vi "LS340Monitor.vi"() -> ()   [LabVIEW 2019]
uses:
  Equipment/Lake Shore Cryotronics 340/Lake Shore Cryotronics 340.lvlib
  Global/Global Variables/Data_Display_global.vi
  Instrument_Setup.vi
panel:
  in  "stop 2":bool
  in  "VISA session 2":refnum<visa-resource-name>="GPIB0::12::INSTR"
  out "SP kleiner als":dbl
  out "Temperature (K)":dbl=291.191
  in  "stop":bool
  in  "VISA session":refnum<visa-resource-name>="GPIB0::12::INSTR"
  out "Temperature":cluster{dbl[], dbl[]}(graph)={[452.667759], [291.191]}
  out "Heater Power":cluster{dbl[], dbl[]}(graph)={[452.667759], [0.0]}
  out "Heater Power (%)":dbl
  out "Heater (%)":dbl(slide) scale=0.0..100.0
  out "Setpoint ITC (K)":dbl=300.0
  out "Offset new SP":dbl
  out "Heater Range":dbl
  out "P (Gain)":dbl
  out "I (Reset)":dbl
  out "D (Rate)":dbl
  in  "Update every [ms]":dbl min=0.0 max=10000.0 step=500.0
  out "HeaterTableLS340.txt":string caption="PID Table"
  in  "Pfad zu HeaterTable":path=path "D:/Cryostat Software/CryoTUM-V1.0/sub_vi-s/Heater Tables/HeaterTableLS340.txt"
  # "0: Off\n1: 10mW\n2: 100mW\n3: 1.0W\n4: 10W"
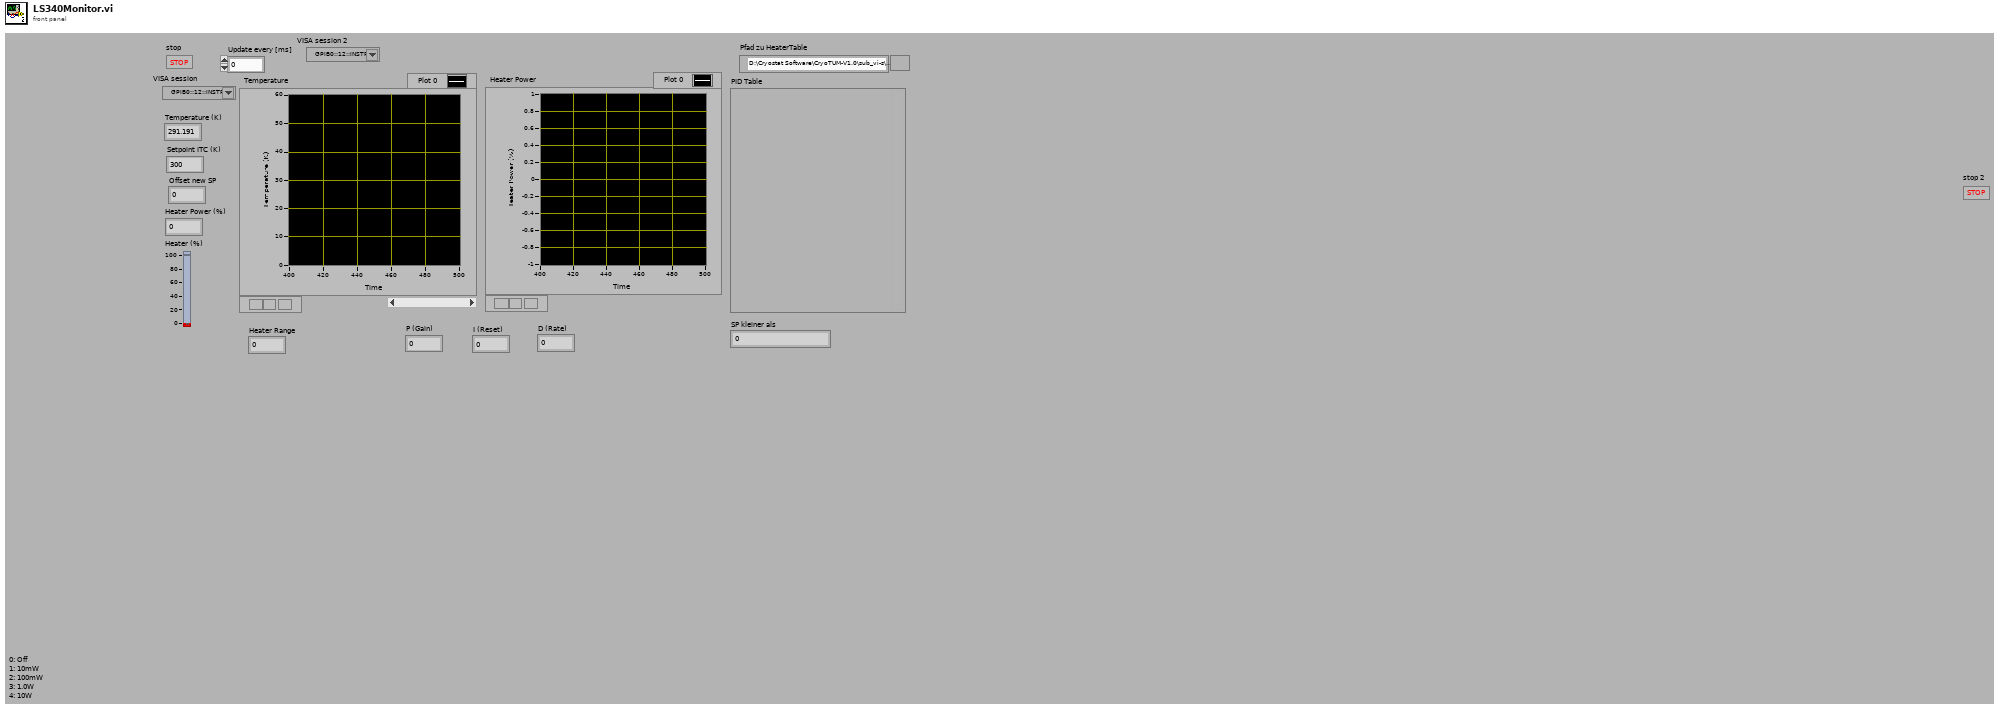
[diagram p1: front panel]
types:
  T1 = enum16{"open", "replace", "create", "open or create", "replace or create", "replace or create with confirmation"}
  T2 = typedef "ITCVersion.ctl" = enum16{"ITC502", "ITC503", "ITC601"}
  T3 = cluster{"Version":T2, "ControlTITC":i8, "ControlTCh":i8, "SampleTITC":i8, "SampleTCh":i8, "Instrument address":cluster{"Com Port":i32, "ISOBUS Address":i32, "GPIB Address":i16, "Communication":enum16{"RS232", "ISOBUS", "GPIB", "Gateway"}}}
  T4 = cluster{"Com Port":i32, "ISOBUS Address":i32, "GPIB Address":i16, "Communication":enum16{"RS232", "ISOBUS", "GPIB", "Gateway"}}
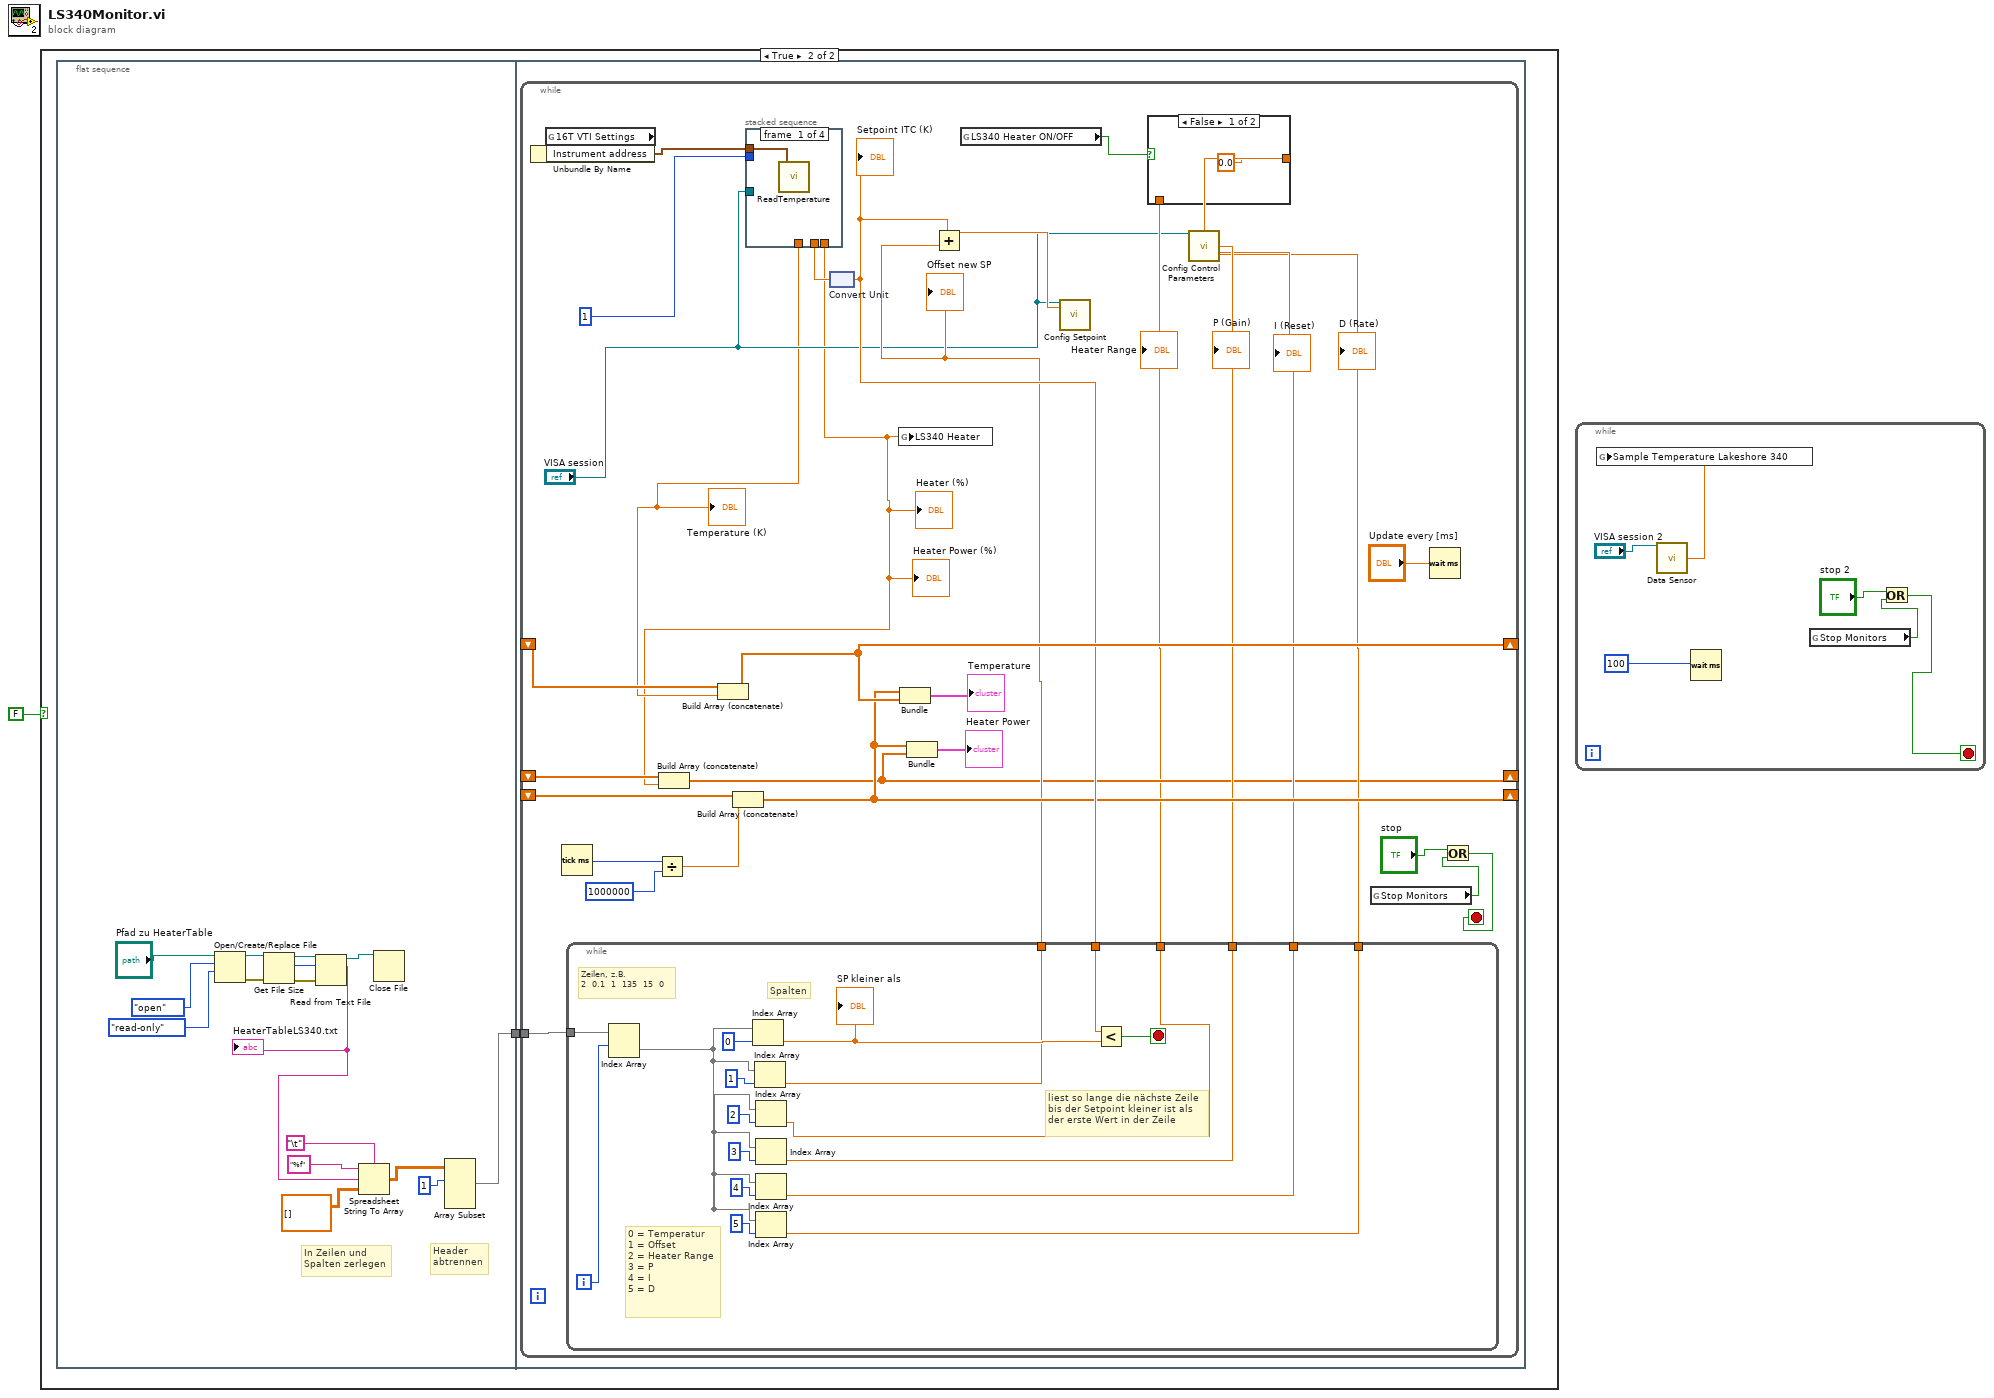
[diagram p0: block diagram]
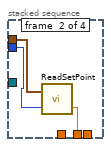
[diagram p3: hidden frame]
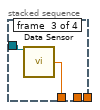
[diagram p4: hidden frame]
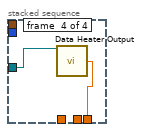
[diagram p5: hidden frame]
diagram:
  n1 = case shown="True" FALSE {
    frame False {
    }
    frame True {
      n2 = flat-sequence {
        tunnel: [w3] -> w2
        tunnel: w2 -> [w19]
        frame #0 {
          # "In Zeilen und \nSpalten zerlegen"
          # "Header\nabtrennen"
          n3 = Open/Create/Replace File(file path (use dialog)="Pfad zu HeaterTable", operation (0:open)=T1."open", access (0:read/write)=enum16{"read/write", "read-only", "write-only"}."read-only") -> (refnum out=w13:refnum<file>, error out=w15:errorcluster)  [unwired: 3 in, 1 out]
          n4 = Get File Size(file=w13, error in=w15) -> (refnum out=w12:refnum<file>, size (in bytes)=w8:i64, 0:w14:errorcluster)
          n5 = Read from Text File(file (use dialog)=w12, count=w8, error in=w14) -> (refnum out=w11:refnum<file>, text=w7:string)  [unwired: 1 in, 2 out]
          "HeaterTableLS340.txt" <- w7
          n6 = Spreadsheet String To Array(delimiter (Tab)="\t", format string="%f", spreadsheet string=w7, array type (2D Dbl)=dbl[][] []) -> (array=w6:dbl[][])
          n7 = Close File(refnum=w11) -> ()  [unwired: 1 in, 2 out]
          n8 = Array Subset(array=w6, index (row)=1) -> (w3:dbl[][])  [unwired: 3 in]
        }
        frame #1 {
          n9 = while {
            shift-right: [w43] -> _
            shift-left: _ -> [w44]
            shift-right: [w33] -> _
            shift-left: _ -> [w51]
            shift-right: [w38] -> _
            shift-left: _ -> [w50]
            tunnel: w19 -> [w41]
            stop <- w28 stop-if-true
            n10 = global read "Instrument_Setup.vi" "16T VTI Settings"() -> (w21:T3)
            n11 = Unbundle By Name(w21) -> ("Instrument address"=w20:T4)
            n12 = Tick Count (ms)() -> (millisecond timer value=w47:u32)
            n13 = Divide(x=w47, y=u32 1000000 ("milliseconds to wait")) -> (x/y=w46:dbl)
            n14 = Build Array (concatenate)(w50, w46) -> (w38:dbl[])
            n15 = stacked-sequence {
              tunnel: w20 -> [w53 w55 _ _]
              tunnel: 1 -> [w52 w54 _ _]
              tunnel: [_ w56 _ _] -> w26
              tunnel: "VISA session" -> [_ _ w58 w60]
              tunnel: [_ _ w57 _] -> w23
              tunnel: [_ _ _ w59] -> w22
              frame #0 {
                n16 = call "ReadTemperature.vi"(6:w52, "IO Info"=w53) -> ()  [unwired: 3 in, 3 out]
              }
              frame #1 {
                n17 = call "ReadSetPoint.vi"("Control Ch"=w54, "IO Info"=w55) -> ("Set point"=w56:dbl[unit])  [unwired: 1 out]
              }
              frame #2 {
                n18 = call "Data Sensor.vi"("VISA resource name"=w58) -> ("Kelvin Reading"=w57:dbl)  [unwired: 10 in, 4 out]
              }
              frame #3 {
                n19 = call "Data Heater Output.vi"("VISA resource name"=w60) -> ("Heater Output"=w59:dbl)  [unwired: 12 in, 2 out]
              }
            }
            "Temperature (K)" <- w23
            "Heater Power (%)" <- w22
            "Heater (%)" <- w22
            n20 = Build Array (concatenate)(w51, w22) -> (w33:dbl[])
            n21 = Build Array (concatenate)(w44, w23) -> (w43:dbl[])
            n22 = node "Convert Unit"(w26) -> (w40:dbl)
            "Setpoint ITC (K)" <- w40
            n23 = while {
              tunnel: w41 -> [w79]
              tunnel: w40 -> [w69]
              tunnel: [w68] -> w37
              tunnel: [w66] -> w32
              tunnel: [w65] -> w36
              tunnel: [w64] -> w35
              tunnel: [w63] -> w34
              i -> [w78]
              stop <- w71 stop-if-true
              # "0 = Temperatur\n1 = Offset\n2 = Heater Range\n3 = P\n4 = I\n5 = D"
              # "liest so lange die nächste Zeile\nbis der Setpoint kleiner ist als \nder erste Wert in der Zeile"
              # "Zeilen, z.B. \n2  0.1  1  135  15  0"
              # "Spalten"
              n24 = Index Array(array=w79, index (row)=w78) -> (element=w72:dbl[])  [unwired: 1 in]
              n25 = Index Array(array=w72, index=0) -> (element=w70:dbl)
              "SP kleiner als" <- w70
              n26 = Index Array(array=w72, index=1) -> (element=w68:dbl)
              n27 = Index Array(array=w72, index=2) -> (element=w66:dbl)
              n28 = Index Array(array=w72, index=3) -> (element=w65:dbl)
              n29 = Index Array(array=w72, index=4) -> (element=w64:dbl)
              n30 = Index Array(array=w72, index=5) -> (element=w63:dbl)
              n31 = Less?(x=w69, y=w70) -> (x < y?=w71:bool)
            }
            "Offset new SP" <- w37
            "Heater Range" <- w32
            "P (Gain)" <- w36
            "I (Reset)" <- w35
            "D (Rate)" <- w34
            n32 = global write "Data_Display_global.vi" "LS340 Heater"(w22) -> ()
            n33 = Bundle(w38, w43) -> (→"Temperature":cluster{dbl[], dbl[]})  [unwired: 1 in]
            n34 = Bundle(w38, w33) -> (→"Heater Power":cluster{dbl[], dbl[]})  [unwired: 1 in]
            n35 = Add(x=w40, y=w37) -> (x+y=w39:dbl)
            n36 = global read "Data_Display_global.vi" "LS340 Heater ON/OFF"() -> (w27:bool)
            n37 = call "Config Setpoint.vi"("VISA resource name"="VISA session", "Setpoint (0.0)"=w39) -> ()  [unwired: 12 in, 2 out]
            n38 = case shown="False" w27 {
              tunnel: w32 -> [_ w62]
              tunnel: [0.0 w62] -> w31
              frame False {
              }
              frame True {
              }
            }
            n39 = call "Config Control Parameters.vi"("VISA resource name"="VISA session", "Heater Range (0: Off)"=w31, "Gain (P) (0.0)"=w36, "Reset (I) (0.0)"=w35, "Rate (D) (0)"=w34) -> ()  [unwired: 9 in, 2 out]
            n40 = global read "Data_Display_global.vi" "Stop Monitors"() -> (w30:bool)
            n41 = Wait (ms)(milliseconds to wait="Update every [ms]") -> ()  [unwired: 1 out]
            n42 = Or(x="stop", y=w30) -> (x .or. y?=w28:bool)
          }
        }
      }
    }
  }
  n43 = while {
    stop <- w81 stop-if-true
    n44 = call "Data Sensor.vi"("VISA resource name"="VISA session 2") -> ("Kelvin Reading"=w84:dbl)  [unwired: 10 in, 4 out]
    n45 = global write "Data_Display_global.vi" "Sample Temperature Lakeshore 340"(w84) -> ()
    n46 = Wait (ms)(milliseconds to wait=u32 100 ("millisecond timer value")) -> ()  [unwired: 1 out]
    n47 = global read "Data_Display_global.vi" "Stop Monitors"() -> (w83:bool)
    n48 = Or(x="stop 2", y=w83) -> (x .or. y?=w81:bool)
  }
